vi "Initiate Measurement.vi"(8 "error in (no error)":errorcluster, 11 "VISA resource name":refnum<visa-resource-name>) -> (0 "error out":errorcluster, 3 "VISA resource name out":refnum<visa-resource-name>)   [LabVIEW 2013, in "Agilent 34401.lvlib"]
doc: "Initiates the measurement according to the instrument model, trigger source, and math configuration.\n\n<B>Note:</B>\n\nThis VI does not check the instrument status. Typically, you call this VI only in a sequence of calls to other low-level instrument driver VIs. The sequence performs one operation. You use the low-level VIs to optimize one or more aspects of interaction with the instrument. If you want to check the instrument status, call the <B>Error Query VI</B> at the conclusion of the sequence."
uses:
  <instrlib>/Agilent 34401/Agilent 34401.lvlib
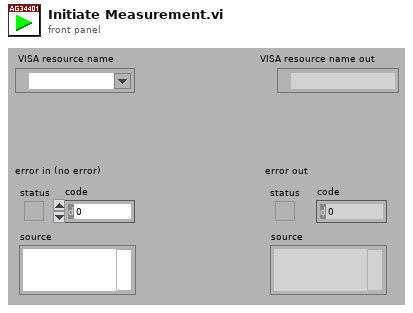
[diagram p1: front panel]
types:
  T1 = typedef "Agilent 34401.lvlib/Extended User Data.ctl" = cluster{"Trigger Source":u16, "Math Storage":u16, "Agilent Model":i32}
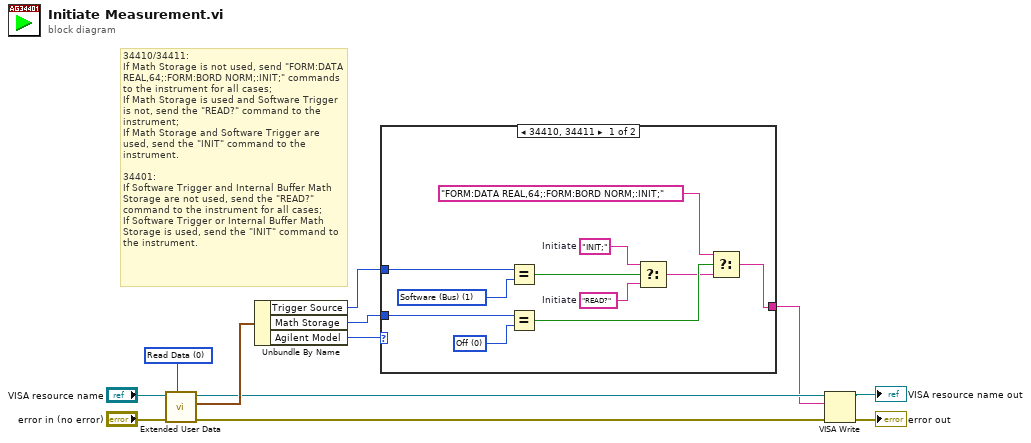
[diagram p0: block diagram]
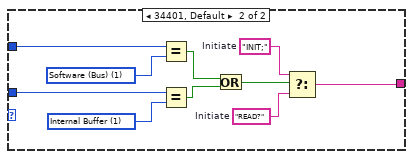
[diagram p2: hidden frame]
diagram:
  w10 = u16 0 items=["Read Data", "Write Data", "Dispose of Data"] ("Action")
  # "34410/34411:\nIf Math Storage is not used, send \"FORM:DATA REAL,64;:FORM:BORD NORM;:INIT;\" commands to the instrument for all cases;\nIf Math Storage is used and Software Trigger is not, send the \"READ?\" command to the instrument;\nIf Math Storage and Software Trigger are used, send the \"INIT\" command to the instrument.\n\n34401:\nIf Software Trigger and Internal Buffer Math Storage are not used, send the \"READ?\" command to the instrument for all cases;\nIf Software Trigger or Internal Buffer Math Storage is used, send the \"INIT\" command to the instrument."
  n1 = call <instrlib>:"Extended User Data.vi"("Action"=w10, "Error In (no error)"="error in (no error)", "VISA resource name in"="VISA resource name") -> ("Error Out"=w3:errorcluster, "User Data Out"=w9:T1, "VISA resource name out"=w2:refnum<visa-resource-name>)  [unwired: 6 in]
  n2 = Unbundle By Name(w9) -> ("Trigger Source"=w7:u16, "Math Storage"=w6:u16, "Agilent Model"=w8:i32)
  n3 = case shown="34410, 34411" w8 {
    tunnel: w6 -> [w19 w28]
    tunnel: w7 -> [w20 w27]
    tunnel: [w18 w26] -> w1
    frame 34410, 34411 {
      w17 = u16 1 items=["Immediate", "Software (Bus)", "External", "Internal"] ("Trigger Source")
      w16 = u16 0 items=["Off", "Internal Buffer", "Output Buffer"] ("Math Storage")
      w23 = "READ?"  # Initiate
      w22 = "INIT;"  # Initiate
      n4 = Equal?(x=w20, y=w17) -> (x = y?=w15:bool)
      n5 = Equal?(x=w19, y=w16) -> (x = y?=w14:bool)
      n6 = Select(t=w22, s=w15, f=w23) -> (s? t:f=w13:string)
      n7 = Select(t="FORM:DATA REAL,64;:FORM:BORD NORM;:INIT;", s=w14, f=w13) -> (s? t:f=w18:string)
    }
    frame 34401, Default {
      w25 = u16 1 items=["Immediate", "Software (Bus)", "External", "Internal"] ("Trigger Source")
      w24 = u16 1 items=["Off", "Internal Buffer", "Output Buffer"] ("Math Storage")
      w30 = "INIT;"  # Initiate
      w29 = "READ?"  # Initiate
      n8 = Equal?(x=w27, y=w25) -> (x = y?=w32:bool)
      n9 = Equal?(x=w28, y=w24) -> (x = y?=w33:bool)
      n10 = Or(x=w32, y=w33) -> (x .or. y?=w31:bool)
      n11 = Select(t=w30, s=w31, f=w29) -> (s? t:f=w26:string)
    }
  }
  n12 = VISA Write(VISA resource name=w2, write buffer=w1, error in (no error)=w3) -> (VISA resource name out=→"VISA resource name out":refnum<visa-resource-name>, error out=→"error out":errorcluster)  [unwired: 1 out]
